vi "Xml_UpdateSupportedTarget.vi"(8 "error in (no error)":errorcluster, 10 "XML String":string="<?xml version=\"1.0\" encoding=\"utf-8\"?>\n<CustomDevice xmlns:xsi=\"http://www.w3.org/2001/XMLSchema-instance\" xsi:noNamespaceSchemaLocation=\"Custom Device.xsd\">\n<XSDVersion Major=\"2010\" Minor=\"0\" Fix=\"0\" Build=\"0\" />\n  <AddMenu>\n    <eng>NI-XNET Monitor</eng>\n    <loc>NI-XNET Monitor</loc>\n  </AddMenu>\n  <Version>2.0.0</Version>\n  <Type>Inline HW Interface</Type>\n  <MaxOccurrence>1</MaxOccurrence>\n  <MainPageGUID>2fba45b0-1589-4179-a966-5fc49498794e</MainPageGUID>\n  <InitializationVI>\n    <Type>Action</Type>\n    <Item2Launch>\n      <Type>To Common Doc Dir</Type>\n\t\t<Path>Custom Devices\\NI-XNET Monitor\\Windows\\NI-XNET Monitor Configuration.llb\\Initialization VI.vi</Path>\n    </Item2Launch>\n  </InitializationVI>\n  <CustomDeviceVI>\n\t\t<SourceDistribution>\n\t\t\t<Source>\n\t\t\t\t<SupportedTarget>Windows</SupportedTarget>\n\t\t\t\t<Source>\n\t\t\t\t\t<Type>To Common Doc Dir</Type>\n\t\t\t\t\t<Path>Custom Devices\\NI-XNET Monitor\\Windows\\NI-XNET Monitor Engine Windows.llb\\RT Driver VI.vi</Path>\n\t\t\t\t</Source>\n\t\t\t\t<RealTimeSystemDestination>c:\\ni-rt\\VeriStand\\Custom Devices\\NI-XNET Monitor\\NI-XNET Monitor Engine Windows.llb\\RT Driver VI.vi</RealTimeSystemDestination>\n\t\t\t</Source>\n\t\t\t<Source>\n\t\t\t\t<SupportedTarget>Pharlap</SupportedTarget>\n\t\t\t\t<Source>\n\t\t\t\t\t<Type>To Common Doc Dir</Type>\n\t\t\t\t\t<Path>Custom Devices\\NI-XNET Monitor\\PharLap\\NI-XNET Monitor Engine Pharlap.llb\\RT Driver VI.vi</Path>\n\t\t\t\t</Source>\n\t\t\t\t<RealTimeSystemDestination>c:\\ni-rt\\VeriStand\\Custom Devices\\NI-XNET Monitor\\NI-XNET Monitor Engine Pharlap.llb\\RT Driver VI.vi</RealTimeSystemDestination>\n\t\t\t</Source>\n\t\t\t<Source>\n\t\t\t\t<SupportedTarget>VxWorks</SupportedTarget>\n\t\t\t\t<Source>\n\t\t\t\t\t<Type>To Common Doc Dir</Type>\n\t\t\t\t\t<Path>Custom Devices\\NI-XNET Monitor\\VxWorks\\NI-XNET Monitor Engine VxWorks.llb\\RT Driver VI.vi</Path>\n\t\t\t\t</Source>\n\t\t\t\t<RealTimeSystemDestination>c:\\ni-rt\\VeriStand\\Custom Devices\\NI-XNET Monitor\\NI-XNET Monitor Engine VxWorks.llb\\RT Driver VI.vi</RealTimeSystemDestination>\n\t\t\t</Source>\t\n\t\t\t<Source>\n\t\t\t\t<SupportedTarget>Linux_32_ARM</SupportedTarget>\n\t\t\t\t<Source>\n\t\t\t\t\t<Type>To Common Doc Dir</Type>\n\t\t\t\t\t<Path>Custom Devices\\NI-XNET Monitor\\Linux_32_ARM\\NI-XNET Monitor Engine LinuxARM.llb\\RT Driver VI.vi</Path>\n\t\t\t\t</Source>\n\t\t\t\t<RealTimeSystemDestination>c:\\ni-rt\\VeriStand\\Custom Devices\\NI-XNET Monitor\\NI-XNET Monitor Engine LinuxARM.llb\\RT Driver VI.vi</RealTimeSystemDestination>\n\t\t\t</Source>\n\t\t\t<Source>\n\t\t\t\t<SupportedTarget>Linux_x64</SupportedTarget>\n\t\t\t\t<Source>\n\t\t\t\t\t<Type>To Common Doc Dir</Type>\n\t\t\t\t\t<Path>Custom Devices\\NI-XNET Monitor\\Linux_x64\\NI-XNET Monitor Engine Linux64.llb\\RT Driver VI.vi</Path>\n\t\t\t\t</Source>\n\t\t\t\t<RealTimeSystemDestination>c:\\ni-rt\\VeriStand\\Custom Devices\\NI-XNET Monitor\\NI-XNET Monitor Engine Linux64.llb\\RT Driver VI.vi</RealTimeSystemDestination>\n\t\t\t</Source>\n\t\t</SourceDistribution>\n\t</CustomDeviceVI>\n  <Dependencies />\n  <Pages>\n    <Page>\n      <Name>\n        <eng>NI-XNET Monitor</eng>\n        <loc>NI-XNET Monitor</loc>\n      </Name>\n\t  <DisallowRenaming>true</DisallowRenaming>\n      <GUID>2fba45b0-1589-4179-a966-5fc49498794e</GUID>\n      <Glyph>\n\t\t\t<Type>To Common Doc Dir</Type>\n\t\t\t<Path>Custom Devices\\NI-XNET Monitor\\Glyphs\\xnet_monitor.png</Path>\n\t\t</Glyph>\n      <Item2Launch>\n        <Type>To Common Doc Dir</Type>\n\t\t<Path>Custom Devices\\NI-XNET Monitor\\Windows\\NI-XNET Monitor Configuration.llb\\Main Page.vi</Path>\n      </Item2Launch>\n\t  <ButtonList>\n\t\t\t<Button>\n\t\t\t\t<ID>Refresh-Button</ID>\n\t\t\t\t<Glyph>\n\t\t\t\t\t<Type>To Application Data Dir</Type>\n\t\t\t\t\t<Path>System Explorer\\Glyphs\\reload.png</Path>\n\t\t\t\t</Glyph>\n\t\t\t\t<Type>Notification</Type>\n\t\t\t\t<ReferencedGUID>2fba45b0-1589-4179-a966-5fc49498794e</ReferencedGUID>\n\t\t\t\t<ButtonText>\n\t\t\t\t\t<eng>Refresh</eng>\n\t\t\t\t\t<loc>Refresh</loc>\n\t\t\t\t</ButtonText>\n\t\t\t\t<Caption>\n\t\t\t\t\t<eng>Refresh</eng>\n\t\t\t\t\t<loc>Refresh</loc>\n\t\t\t\t</Caption>\n\t\t\t\t<TipStrip>\n\t\t\t\t\t<eng>Refresh NI-XNET channel list</eng>\n\t\t\t\t\t<loc>Refresh NI-XNET channel list</loc>\n\t\t\t\t</TipStrip>\n\t\t\t\t<Documentation>\n\t\t\t\t\t<eng>Refresh NI-XNET channel list</eng>\n\t\t\t\t\t<loc>Refresh NI-XNET channel list</loc>\n\t\t\t\t</Documentation>\n\t\t\t</Button>\n\t  </ButtonList>\n\t  <ActionVIOnDelete>\n \t\t <Type>To Common Doc Dir</Type>\n\t\t <Path>Custom Devices\\NI-XNET Monitor\\Windows\\NI-XNET Monitor Configuration.llb\\ActionVIOnDelete.vi</Path>\n\t  </ActionVIOnDelete>\n      <ActionVIOnLoad>\n        <Type>To Common Doc Dir</Type>\n        <Path>Custom Devices\\NI-XNET Monitor\\Windows\\NI-XNET Monitor Configuration.llb\\ActionVIOnLoad.vi</Path>\n      </ActionVIOnLoad>\n      <ActionVIOnSave>\n        <Type>To Common Doc Dir</Type>\n        <Path>Custom Devices\\NI-XNET Monitor\\Windows\\NI-XNET Monitor Configuration.llb\\ActionVIOnSave.vi</Path>\n      </ActionVIOnSave>\n\t  <ActionVIOnCompile>\n        <Type>To Common Doc Dir</Type>\n        <Path>Custom Devices\\NI-XNET Monitor\\Windows\\NI-XNET Monitor Configuration.llb\\ActionVIOnCompile.vi</Path>\n      </ActionVIOnCompile>\n    </Page>\n    \n<Page>\n      <Name>\n        <eng>Port</eng>\n        <loc>Port</loc>\n      </Name>\n\t  <DisallowRenaming>true</DisallowRenaming>\n\t  <ExcludeFromAlphabeticalOrder>true</ExcludeFromAlphabeticalOrder>\n      <GUID>6e4b4e9f-3d48-4140-aa73-eb1a9ddd4810</GUID>\n      <Glyph>\n\t\t\t<Type>To Application Data Dir</Type>\n\t\t\t<Path>System Explorer\\Glyphs\\NI-XNET Port.png</Path>\n\t\t</Glyph>\n      <Item2Launch>\n        <Type>To Common Doc Dir</Type>\n\t\t<Path>Custom Devices\\NI-XNET Monitor\\Windows\\NI-XNET Monitor Configuration.llb\\Port.vi</Path>\n      </Item2Launch>\n\t  <ButtonList>\n\t\t\t<Button>\n\t\t\t\t<ID>Refresh-Button</ID>\n\t\t\t\t<Glyph>\n\t\t\t\t\t<Type>To Application Data Dir</Type>\n\t\t\t\t\t<Path>System Explorer\\Glyphs\\reload.png</Path>\n\t\t\t\t</Glyph>\n\t\t\t\t<Type>Notification</Type>\n\t\t\t\t<ReferencedGUID>6e4b4e9f-3d48-4140-aa73-eb1a9ddd4810</ReferencedGUID>\n\t\t\t\t<ButtonText>\n\t\t\t\t\t<eng>Refresh</eng>\n\t\t\t\t\t<loc>Refresh</loc>\n\t\t\t\t</ButtonText>\n\t\t\t\t<Caption>\n\t\t\t\t\t<eng>Refresh</eng>\n\t\t\t\t\t<loc>Refresh</loc>\n\t\t\t\t</Caption>\n\t\t\t\t<TipStrip>\n\t\t\t\t\t<eng>Refresh NI-XNET channel list</eng>\n\t\t\t\t\t<loc>Refresh NI-XNET channel list</loc>\n\t\t\t\t</TipStrip>\n\t\t\t\t<Documentation>\n\t\t\t\t\t<eng>Refresh NI-XNET channel list</eng>\n\t\t\t\t\t<loc>Refresh NI-XNET channel list</loc>\n\t\t\t\t</Documentation>\n\t\t\t</Button>\n\t  </ButtonList>\n    </Page>\n<Page>\n      <Name>\n        <eng>Port</eng>\n        <loc>Port</loc>\n      </Name>\n\t  <DisallowRenaming>true</DisallowRenaming>\n\t  <ExcludeFromAlphabeticalOrder>true</ExcludeFromAlphabeticalOrder>\n      <GUID>6e4b4e9f-3d48-4140-aa73-eb1a9ddd4810-DISABLED</GUID>\n      <Glyph>\n\t\t\t<Type>To Application Data Dir</Type>\n\t\t\t<Path>System Explorer\\Glyphs\\NI-XNET Port Disabled.png</Path>\n\t\t</Glyph>\n      <Item2Launch>\n        <Type>To Common Doc Dir</Type>\n\t\t<Path>Custom Devices\\NI-XNET Monitor\\Windows\\NI-XNET Monitor Configuration.llb\\Port.vi</Path>\n      </Item2Launch>\n\t  <ButtonList>\n\t\t\t<Button>\n\t\t\t\t<ID>Refresh-Button</ID>\n\t\t\t\t<Glyph>\n\t\t\t\t\t<Type>To Application Data Dir</Type>\n\t\t\t\t\t<Path>System Explorer\\Glyphs\\reload.png</Path>\n\t\t\t\t</Glyph>\n\t\t\t\t<Type>Notification</Type>\n\t\t\t\t<ReferencedGUID>6e4b4e9f-3d48-4140-aa73-eb1a9ddd4810-DISABLED</ReferencedGUID>\n\t\t\t\t<ButtonText>\n\t\t\t\t\t<eng>Refresh</eng>\n\t\t\t\t\t<loc>Refresh</loc>\n\t\t\t\t</ButtonText>\n\t\t\t\t<Caption>\n\t\t\t\t\t<eng>Refresh</eng>\n\t\t\t\t\t<loc>Refresh</loc>\n\t\t\t\t</Caption>\n\t\t\t\t<TipStrip>\n\t\t\t\t\t<eng>Refresh NI-XNET channel list</eng>\n\t\t\t\t\t<loc>Refresh NI-XNET channel list</loc>\n\t\t\t\t</TipStrip>\n\t\t\t\t<Documentation>\n\t\t\t\t\t<eng>Refresh NI-XNET channel list</eng>\n\t\t\t\t\t<loc>Refresh NI-XNET channel list</loc>\n\t\t\t\t</Documentation>\n\t\t\t</Button>\n\t  </ButtonList>\n    </Page>\n<Page>\n      <Name>\n        <eng>CAN</eng>\n        <loc>CAN</loc>\n      </Name>\n\t  <DisallowRenaming>true</DisallowRenaming>\n\t  <ExcludeFromAlphabeticalOrder>true</ExcludeFromAlphabeticalOrder>\n      <GUID>d0ed4327-8d71-4af7-8daf-159d159a2198</GUID>\n      <Glyph>\n\t\t\t<Type>To Application Data Dir</Type>\n\t\t\t<Path>System Explorer\\Glyphs\\NI-XNET CAN.png</Path>\n\t\t</Glyph>\n      <Item2Launch>\n        <Type>To Common Doc Dir</Type>\n\t\t<Path>Custom Devices\\NI-XNET Monitor\\Windows\\NI-XNET Monitor Configuration.llb\\Interface.vi</Path>\n      </Item2Launch>\n\t  <ButtonList>\n\t\t\t<Button>\n\t\t\t\t<ID>Refresh-Button</ID>\n\t\t\t\t<Glyph>\n\t\t\t\t\t<Type>To Application Data Dir</Type>\n\t\t\t\t\t<Path>System Explorer\\Glyphs\\reload.png</Path>\n\t\t\t\t</Glyph>\n\t\t\t\t<Type>Notification</Type>\n\t\t\t\t<ReferencedGUID>d0ed4327-8d71-4af7-8daf-159d159a2198</ReferencedGUID>\n\t\t\t\t<ButtonText>\n\t\t\t\t\t<eng>Refresh</eng>\n\t\t\t\t\t<loc>Refresh</loc>\n\t\t\t\t</ButtonText>\n\t\t\t\t<Caption>\n\t\t\t\t\t<eng>Refresh</eng>\n\t\t\t\t\t<loc>Refresh</loc>\n\t\t\t\t</Caption>\n\t\t\t\t<TipStrip>\n\t\t\t\t\t<eng>Refresh NI-XNET channel list</eng>\n\t\t\t\t\t<loc>Refresh NI-XNET channel list</loc>\n\t\t\t\t</TipStrip>\n\t\t\t\t<Documentation>\n\t\t\t\t\t<eng>Refresh NI-XNET channel list</eng>\n\t\t\t\t\t<loc>Refresh NI-XNET channel list</loc>\n\t\t\t\t</Documentation>\n\t\t\t</Button>\n\t  </ButtonList>\n    </Page>\n<Page>\n      <Name>\n        <eng>FlexRay</eng>\n        <loc>FlexRay</loc>\n      </Name>\n\t  <DisallowRenaming>true</DisallowRenaming>\n\t  <ExcludeFromAlphabeticalOrder>true</ExcludeFromAlphabeticalOrder>\n      <GUID>b3b15e68-7151-4c2d-a280-06a82878b967</GUID>\n      <Glyph>\n\t\t\t<Type>To Application Data Dir</Type>\n\t\t\t<Path>System Explorer\\Glyphs\\NI-XNET FlexRay.png</Path>\n\t\t</Glyph>\n      <Item2Launch>\n        <Type>To Common Doc Dir</Type>\n\t\t<Path>Custom Devices\\NI-XNET Monitor\\Windows\\NI-XNET Monitor Configuration.llb\\Interface.vi</Path>\n      </Item2Launch>\n\t  <ButtonList>\n\t\t\t<Button>\n\t\t\t\t<ID>Refresh-Button</ID>\n\t\t\t\t<Glyph>\n\t\t\t\t\t<Type>To Application Data Dir</Type>\n\t\t\t\t\t<Path>System Explorer\\Glyphs\\reload.png</Path>\n\t\t\t\t</Glyph>\n\t\t\t\t<Type>Notification</Type>\n\t\t\t\t<ReferencedGUID>b3b15e68-7151-4c2d-a280-06a82878b967</ReferencedGUID>\n\t\t\t\t<ButtonText>\n\t\t\t\t\t<eng>Refresh</eng>\n\t\t\t\t\t<loc>Refresh</loc>\n\t\t\t\t</ButtonText>\n\t\t\t\t<Caption>\n\t\t\t\t\t<eng>Refresh</eng>\n\t\t\t\t\t<loc>Refresh</loc>\n\t\t\t\t</Caption>\n\t\t\t\t<TipStrip>\n\t\t\t\t\t<eng>Refresh NI-XNET channel list</eng>\n\t\t\t\t\t<loc>Refresh NI-XNET channel list</loc>\n\t\t\t\t</TipStrip>\n\t\t\t\t<Documentation>\n\t\t\t\t\t<eng>Refresh NI-XNET channel list</eng>\n\t\t\t\t\t<loc>Refresh NI-XNET channel list</loc>\n\t\t\t\t</Documentation>\n\t\t\t</Button>\n\t  </ButtonList>\n    </Page>\n<Page>\n      <Name>\n        <eng>LIN</eng>\n        <loc>LIN</loc>\n      </Name>\n\t  <DisallowRenaming>true</DisallowRenaming>\n\t  <ExcludeFromAlphabeticalOrder>true</ExcludeFromAlphabeticalOrder>\n      <GUID>c19a2e81-5516-4045-93a5-b1bca7ac20ae</GUID>\n      <Glyph>\n\t\t\t<Type>To Application Data Dir</Type>\n\t\t\t<Path>System Explorer\\Glyphs\\NI-XNET LIN.png</Path>\n\t\t</Glyph>\n      <Item2Launch>\n        <Type>To Common Doc Dir</Type>\n\t\t<Path>Custom Devices\\NI-XNET Monitor\\Windows\\NI-XNET Monitor Configuration.llb\\Interface.vi</Path>\n      </Item2Launch>\n\t  <ButtonList>\n\t\t\t<Button>\n\t\t\t\t<ID>Refresh-Button</ID>\n\t\t\t\t<Glyph>\n\t\t\t\t\t<Type>To Application Data Dir</Type>\n\t\t\t\t\t<Path>System Explorer\\Glyphs\\reload.png</Path>\n\t\t\t\t</Glyph>\n\t\t\t\t<Type>Notification</Type>\n\t\t\t\t<ReferencedGUID>c19a2e81-5516-4045-93a5-b1bca7ac20ae</ReferencedGUID>\n\t\t\t\t<ButtonText>\n\t\t\t\t\t<eng>Refresh</eng>\n\t\t\t\t\t<loc>Refresh</loc>\n\t\t\t\t</ButtonText>\n\t\t\t\t<Caption>\n\t\t\t\t\t<eng>Refresh</eng>\n\t\t\t\t\t<loc>Refresh</loc>\n\t\t\t\t</Caption>\n\t\t\t\t<TipStrip>\n\t\t\t\t\t<eng>Refresh NI-XNET channel list</eng>\n\t\t\t\t\t<loc>Refresh NI-XNET channel list</loc>\n\t\t\t\t</TipStrip>\n\t\t\t\t<Documentation>\n\t\t\t\t\t<eng>Refresh NI-XNET channel list</eng>\n\t\t\t\t\t<loc>Refresh NI-XNET channel list</loc>\n\t\t\t\t</Documentation>\n\t\t\t</Button>\n\t  </ButtonList>\n    </Page>\n<Page>\n      <Name>\n        <eng>PortStatus</eng>\n        <loc>PortStatus</loc>\n      </Name>\n\t  <DisallowRenaming>true</DisallowRenaming>\n\t  <ExcludeFromAlphabeticalOrder>true</ExcludeFromAlphabeticalOrder>\n      <GUID>20dbf2c1-039f-4944-a9cd-53b00268baa8</GUID>\n      <Glyph>\n\t\t\t<Type>To Application Data Dir</Type>\n\t\t\t<Path>System Explorer\\Glyphs\\system variable.png</Path>\n\t\t</Glyph>\n      <Item2Launch>\n        <Type>To Common Doc Dir</Type>\n\t\t<Path>Custom Devices\\NI-XNET Monitor\\Windows\\NI-XNET Monitor Configuration.llb\\PortChannel.vi</Path>\n      </Item2Launch>\n    </Page>\n<Page>\n      <Name>\n        <eng>PortError</eng>\n        <loc>PortError</loc>\n      </Name>\n\t  <DisallowRenaming>true</DisallowRenaming>\n\t  <ExcludeFromAlphabeticalOrder>true</ExcludeFromAlphabeticalOrder>\n      <GUID>37c19a15-61f7-4078-98c8-bfb7f6b25de3</GUID>\n      <Glyph>\n\t\t\t<Type>To Application Data Dir</Type>\n\t\t\t<Path>System Explorer\\Glyphs\\NI-XNET TransceiverState.png</Path>\n\t\t</Glyph>\n      <Item2Launch>\n        <Type>To Common Doc Dir</Type>\n\t\t<Path>Custom Devices\\NI-XNET Monitor\\Windows\\NI-XNET Monitor Configuration.llb\\PortChannel.vi</Path>\n      </Item2Launch>\n    </Page>\n  </Pages>\n  <CustomXML>\n    <Dummy></Dummy>\n  </CustomXML>\n</CustomDevice>", 11 "XML Path":path=path "\\\\vmware-host\\Shared Folders/_Repo/NI-XNET-Monitor-Custom-Device/Source/Custom Device NI-XNET Monitor.xml") -> (0 "error out":errorcluster)   [LabVIEW 2020, in "Shared.lvlib"]
uses:
  Shared.lvlib
  <vilib>/xml/Load XML String.vi
  <vilib>/xml/Close Reference(Node).vi
  <vilib>/xml/NI_XML.lvlib
  <resource>/objmgr/DOMUserDefRef.rc
panel:
  out "XML":string
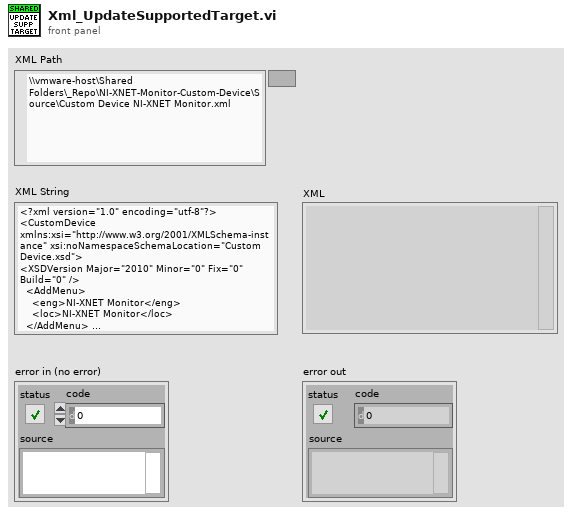
[diagram p1: front panel]
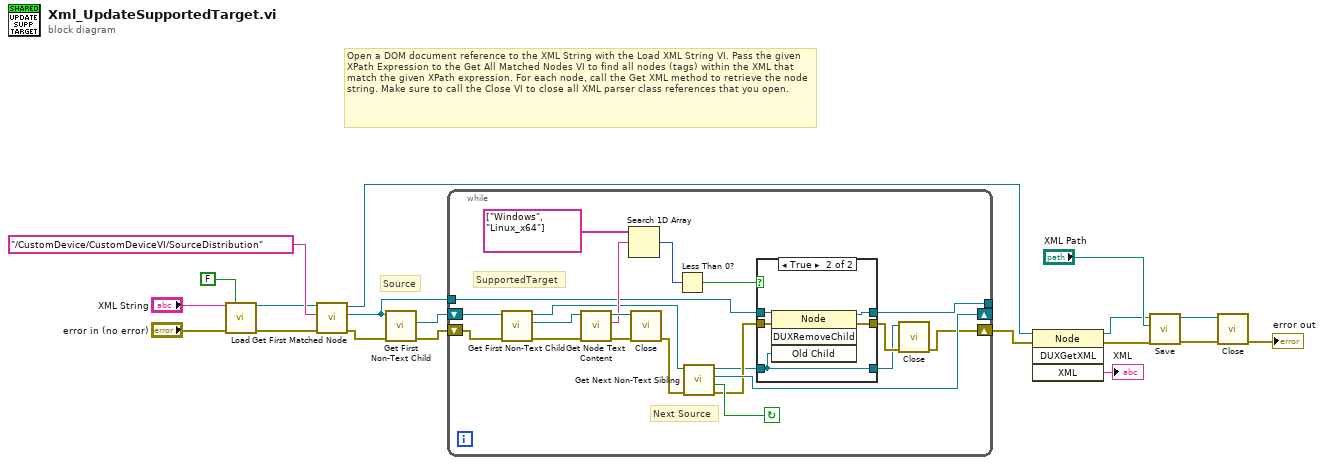
[diagram p0: block diagram]
diagram:
  # "Source"
  # "Open a DOM document reference to the XML String with the Load XML String VI. Pass the given XPath Expression to the Get All Matched Nodes VI to find all nodes (tags) within the XML that match the given XPath expression. For each node, call the Get XML method to retrieve the node string. Make sure to call the Close VI to close all XML parser class references that you open."
  n1 = call-poly <vilib>:"Load.vi"("XML string"="XML String", "preserve whitespace (True)"=FALSE, "error in (no error)"="error in (no error)") -> ("DOM document out"=w8:refnum<k20>, "error out"=w19:errorcluster)  [unwired: 10 in, 1 out]
  n2 = call <vilib>:"Get First Matched Node.vi"("error in (no error)"=w19, "XPath expression"="/CustomDevice/CustomDeviceVI/SourceDistribution" ("XPath Expression"), "node in"=w8) -> ("error out"=w15:errorcluster, "node result"=w13:refnum<k20>, "node out"=w9:refnum<k20>)  [unwired: 6 in]
  n3 = call <vilib>:"Get First Non-Text Child.vi"("error in (no error)"=w15, "node in"=w13) -> ("error out"=w14:errorcluster, "child node"=w10:refnum<k20>)  [unwired: 6 in, 2 out]
  n4 = while {
    tunnel: w13 -> [w22]
    shift-right: [w30] -> _
    shift-left: w10 -> [w21]
    shift-right: [w26] -> w11
    shift-left: w14 -> [w32]
    tunnel: [w33] -> _
    stop <- w29 continue-if-true
    # "Next Source"
    # "SupportedTarget"
    n5 = call <vilib>:"Get First Non-Text Child.vi"("error in (no error)"=w32, "node in"=w21) -> ("error out"=w37:errorcluster, "child node"=w38:refnum<k20>, "node out"=w24:refnum<k20>)  [unwired: 6 in, 1 out]
    n6 = call <vilib>:"Get Node Text Content.vi"("error in (no error)"=w37, "node in"=w38) -> ("error out"=w40:errorcluster, "node text"=w35:string, "node out"=w39:refnum<k20>)  [unwired: 7 in]
    n7 = Search 1D Array(1D array=string[] ["Windows", "Linux_x64"], element=w35) -> (index of element=w34:i32)  [unwired: 1 in]
    n8 = call-poly <vilib>:"Close.vi"("error in (no error)"=w40, "node"=w39) -> ("error out"=w31:errorcluster)  [unwired: 7 out]
    n9 = Less Than 0?(x=w34) -> (x < 0?=w20:bool)
    n10 = call <vilib>:"Get Next Non-Text Sibling.vi"("error in (no error)"=w31, "node in"=w24) -> ("error out"=w28:errorcluster, "found sibling node?"=w29:bool, "sibling node"=w30:refnum<k20>, "node out"=w23:refnum<k20>)  [unwired: 6 in]
    n11 = case shown="True" w20 {
      tunnel: w22 -> [w43 w48]
      tunnel: w23 -> [w41 w44]
      tunnel: w28 -> [w42 w47]
      tunnel: [w43 w46] -> w33
      tunnel: [w42 w45] -> w27
      tunnel: [w41 w44] -> w25
      frame False {
      }
      frame True {
        n12 = invoke class="Node" method="DUXRemoveChild"(reference=w48, error in=w47, "Old Child"=w44) -> (reference out=w46:refnum<k20>, error out=w45:errorcluster)  [unwired: 1 in, 2 out]
      }
    }
    n13 = call-poly <vilib>:"Close.vi"("error in (no error)"=w27, "node"=w25) -> ("error out"=w26:errorcluster)  [unwired: 7 out]
  }
  n14 = invoke class="Node" method="DUXGetXML"(reference=w9, error in=w11) -> (reference out=w6:refnum<k20>, error out=w5:errorcluster, "XML"=→"XML":string)  [unwired: 2 in, 1 out]
  n15 = call <vilib>:"Save.vi"("error in (no error)"=w5, "XML file path"="XML Path", "DOM document in"=w6) -> ("error out"=w3:errorcluster, "DOM document out"=w4:refnum<k20>)  [unwired: 6 in, 1 out]
  n16 = call-poly <vilib>:"Close.vi"("error in (no error)"=w3, "node"=w4) -> ("error out"=→"error out":errorcluster)  [unwired: 7 out]
